vi "Rolling Display.vi"(6 "Input Data":dbl[][](array[numeric]), 9 "Old Data":dbl[][](array[numeric]), 10 "Sample Rate":i32, 11 "Display Size":T3(ring)) -> ()   [LabVIEW 2014]
panel:
  out "Cluster":T1
  in  "Channels in Use":T2
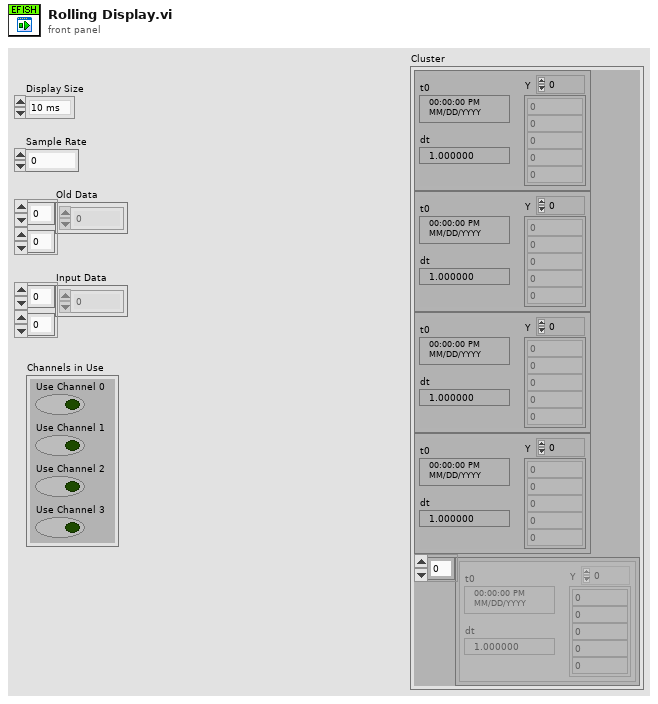
[diagram p1: front panel]
types:
  T1 = cluster{"Waveform":waveform(dbl), "Waveform":waveform(dbl), "Waveform":waveform(dbl), "Waveform":waveform(dbl), waveform(dbl)[]}
  T2 = cluster{"Use Channel 0":bool, "Use Channel 1":bool, "Use Channel 2":bool, "Use Channel 3":bool}
  T3 = enum16{"10 ms", "100 ms", "1 Second", "10 sec", "30 sec"}
  T4 = cluster{waveform(dbl), waveform(dbl), waveform(dbl), waveform(dbl), waveform(dbl)[]}
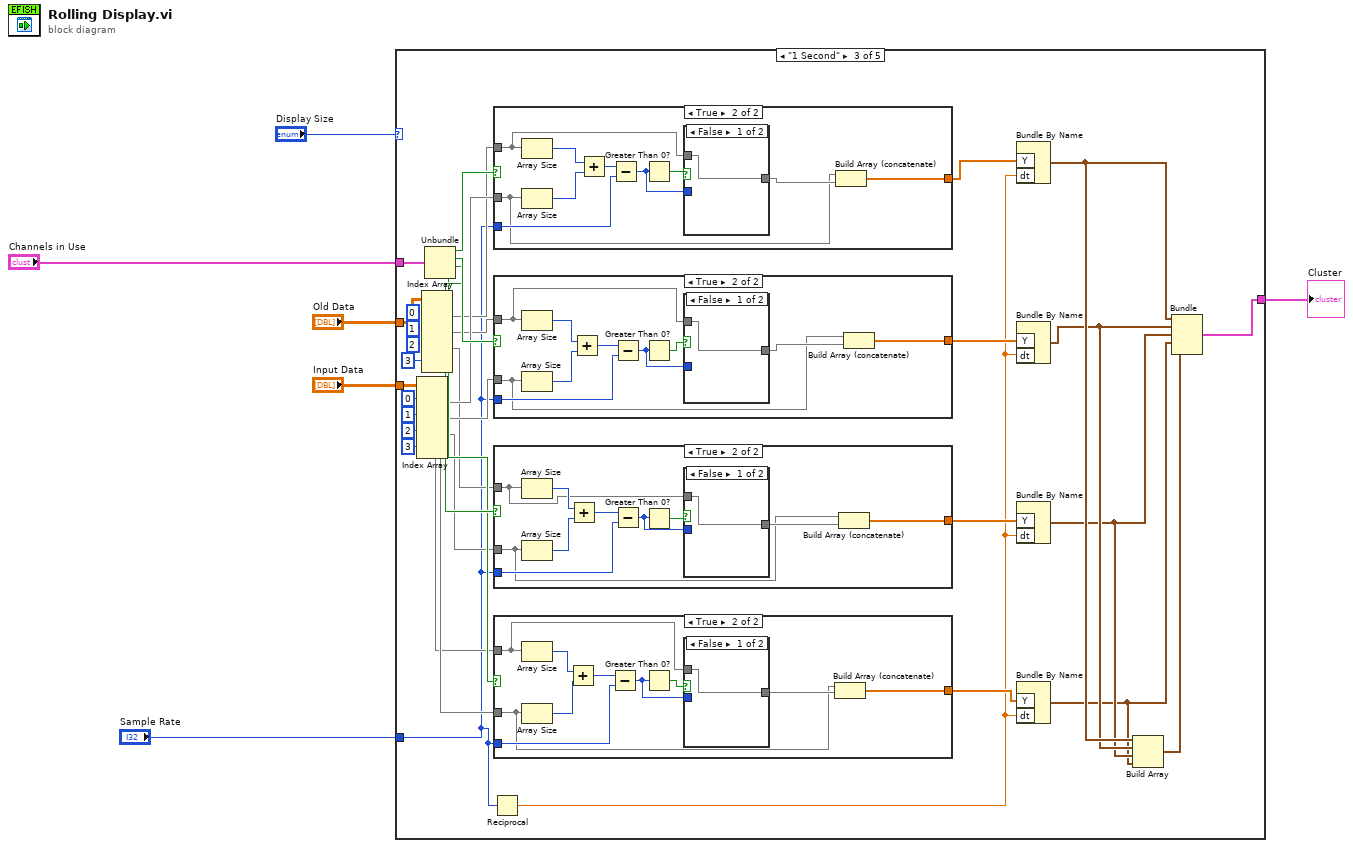
[diagram p0: block diagram]
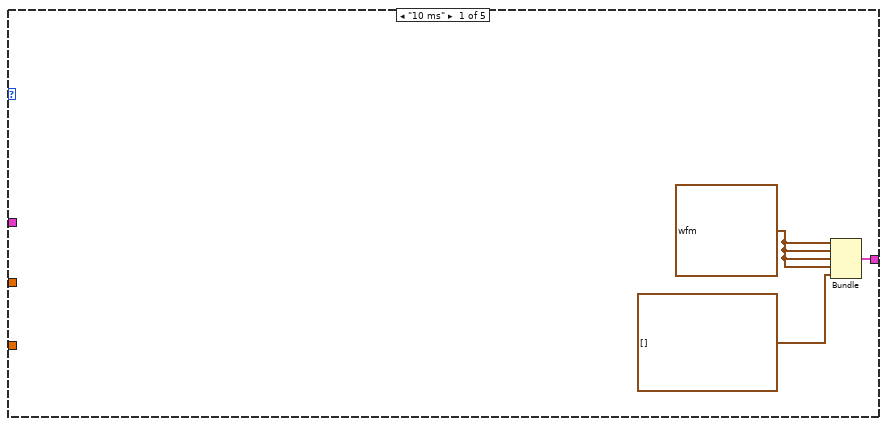
[diagram p2: hidden frame]
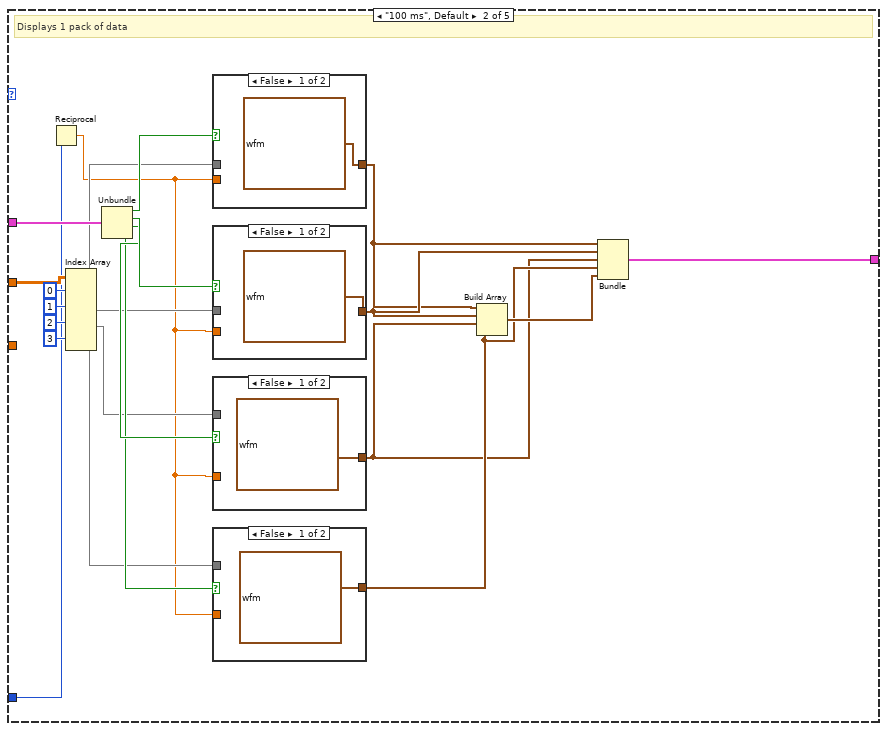
[diagram p3: hidden frame]
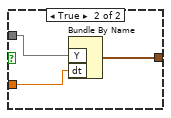
[diagram p4: hidden frame]
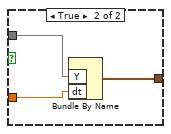
[diagram p5: hidden frame]
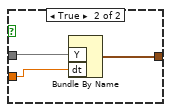
[diagram p6: hidden frame]
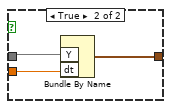
[diagram p7: hidden frame]
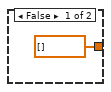
[diagram p8: hidden frame]
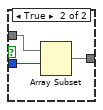
[diagram p9: hidden frame]
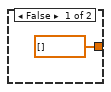
[diagram p10: hidden frame]
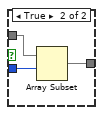
[diagram p11: hidden frame]
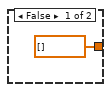
[diagram p12: hidden frame]
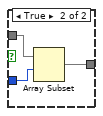
[diagram p13: hidden frame]
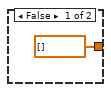
[diagram p14: hidden frame]
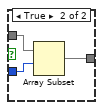
[diagram p15: hidden frame]
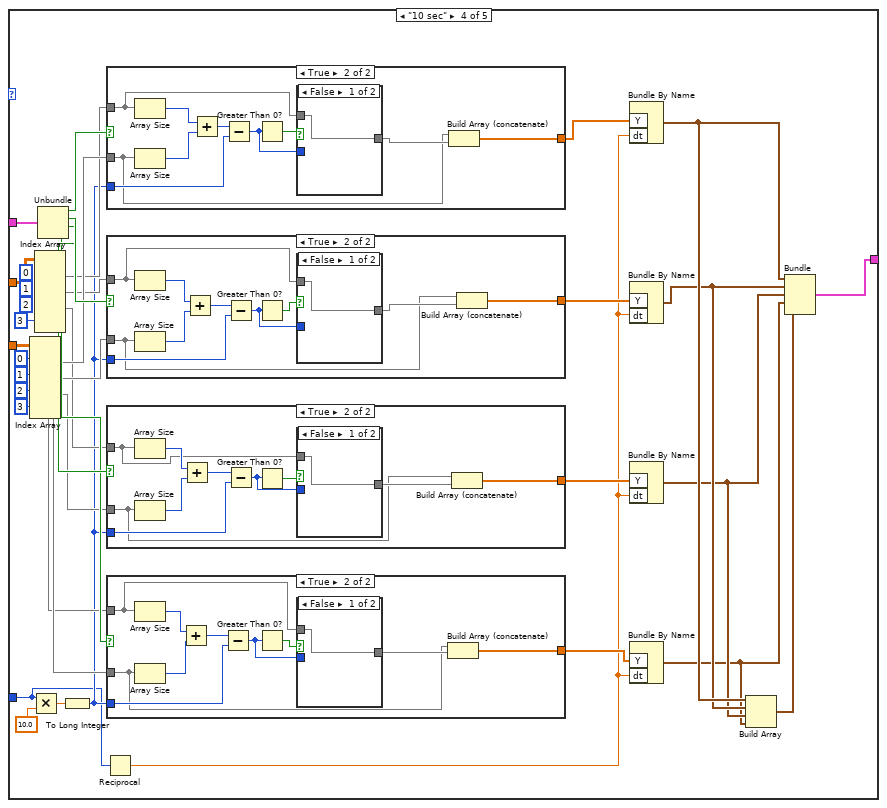
[diagram p16: hidden frame]
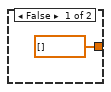
[diagram p17: hidden frame]
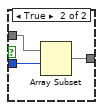
[diagram p18: hidden frame]
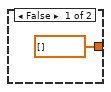
[diagram p19: hidden frame]
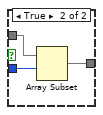
[diagram p20: hidden frame]
diagram:
  n1 = case shown="\"1 Second\"" "Display Size" {
    tunnel: "Sample Rate" -> [_ w17 w48 w147 w242]
    tunnel: "Input Data" -> [_ _ w74 w169 w264]
    tunnel: "Old Data" -> [_ w26 w64 w159 w254]
    tunnel: "Channels in Use" -> [_ w31 w79 w174 w269]
    tunnel: [w9 w10 w49 w140 w235] -> w1
    frame "10 ms" {
      w8 = waveform(dbl) {"t0"=timestamp(0 s since 1904-01-01), "dt"=1.0, "Y"=[]}
      n2 = Bundle(w8, w8, w8, w8, waveform(dbl)[] []) -> (w9:T4)  [unwired: 1 in]
    }
    frame "100 ms", Default {
      # "Displays 1 pack of data"
      n3 = Reciprocal(x=w17) -> (1/x=w16:dbl)
      n4 = Index Array(array=w26, index (row) #1=0 ("index (row)"), index (row) #2=1 ("index (row)"), index (row) #3=2 ("index (row)"), index (row) #4=3 ("index (row)")) -> (element #1=w21:dbl[], element #2=w20:dbl[], element #3=w19:dbl[], element #4=w18:dbl[])  [unwired: 4 in]
      n5 = Unbundle(w31) -> ("Use Channel 0"=w30:bool, "Use Channel 1"=w29:bool, "Use Channel 2"=w28:bool, "Use Channel 3"=w27:bool)
      n6 = case shown="False" w30 {
        tunnel: w21 -> [_ w47]
        tunnel: w16 -> [_ w46]
        tunnel: [waveform(dbl) {"t0"=timestamp(0 s since 1904-01-01), "dt"=1.0, "Y"=[]} w45] -> w11
        frame False {
        }
        frame True {
          n7 = Bundle By Name("Y"=w47, "dt"=w46) -> (w45:waveform(dbl))  [unwired: 1 in]
        }
      }
      n8 = case shown="False" w29 {
        tunnel: w20 -> [_ w43]
        tunnel: w16 -> [_ w42]
        tunnel: [waveform(dbl) {"t0"=timestamp(0 s since 1904-01-01), "dt"=1.0, "Y"=[]} w41] -> w12
        frame False {
        }
        frame True {
          n9 = Bundle By Name("Y"=w43, "dt"=w42) -> (w41:waveform(dbl))  [unwired: 1 in]
        }
      }
      n10 = case shown="False" w28 {
        tunnel: w19 -> [_ w38]
        tunnel: w16 -> [_ w39]
        tunnel: [waveform(dbl) {"t0"=timestamp(0 s since 1904-01-01), "dt"=1.0, "Y"=[]} w37] -> w13
        frame False {
        }
        frame True {
          n11 = Bundle By Name("Y"=w38, "dt"=w39) -> (w37:waveform(dbl))  [unwired: 1 in]
        }
      }
      n12 = case shown="False" w27 {
        tunnel: w18 -> [_ w35]
        tunnel: w16 -> [_ w34]
        tunnel: [waveform(dbl) {"t0"=timestamp(0 s since 1904-01-01), "dt"=1.0, "Y"=[]} w33] -> w14
        frame False {
        }
        frame True {
          n13 = Bundle By Name("Y"=w35, "dt"=w34) -> (w33:waveform(dbl))  [unwired: 1 in]
        }
      }
      n14 = Build Array(w11, w12, w13, w14) -> (w15:waveform(dbl)[])
      n15 = Bundle(w11, w12, w13, w14, w15) -> (w10:T4)  [unwired: 1 in]
    }
    frame "1 Second" {
      (unwired) 2 ("index (row)")
      (unwired) 1 ("index (row)")
      (unwired) 0 ("index (row)")
      n16 = Index Array(array=w74, index (row) #1=0 ("index (row)"), index (row) #2=1 ("index (row)"), index (row) #3=2 ("index (row)"), index (row) #4=3 ("index (row)")) -> (element #1=w69:dbl[], element #2=w68:dbl[], element #3=w67:dbl[], element #4=w66:dbl[])  [unwired: 4 in]
      n17 = Index Array(array=w64, index (row) #4=3 ("index (row)")) -> (element #1=w63:dbl[], element #2=w62:dbl[], element #3=w61:dbl[], element #4=w60:dbl[])  [unwired: 7 in]
      n18 = Unbundle(w79) -> ("Use Channel 0"=w78:bool, "Use Channel 1"=w77:bool, "Use Channel 2"=w76:bool, "Use Channel 3"=w75:bool)
      n19 = Reciprocal(x=w48) -> (1/x=w55:dbl)
      n20 = case shown="True" w78 {
        tunnel: w69 -> [_ w127]
        tunnel: w63 -> [_ w129]
        tunnel: w48 -> [_ w132]
        tunnel: [dbl[] [] w126] -> w59
        frame False {
        }
        frame True {
          n21 = Array Size(array=w129) -> (size(s)=w135:i32)
          n22 = Array Size(array=w127) -> (size(s)=w134:i32)
          n23 = Add(x=w135, y=w134) -> (x+y=w133:i32)
          n24 = Subtract(x=w133, y=w132) -> (x-y=w130:i32)
          n25 = Greater Than 0?(x=w130) -> (x > 0?=w131:bool)
          n26 = case shown="False" w131 {
            tunnel: w130 -> [_ w139]
            tunnel: w129 -> [w136 w138]
            tunnel: [w136 w137] -> w128
            frame False {
            }
            frame True {
              n27 = Array Subset(array=w138, index=w139) -> (w137:dbl[])  [unwired: 1 in]
            }
          }
          n28 = Build Array (concatenate)(w127, w128) -> (w126:dbl[])
        }
      }
      n29 = case shown="True" w77 {
        tunnel: w68 -> [_ w112]
        tunnel: w62 -> [_ w114]
        tunnel: w48 -> [_ w117]
        tunnel: [dbl[] [] w111] -> w58
        frame False {
        }
        frame True {
          n30 = Array Size(array=w114) -> (size(s)=w120:i32)
          n31 = Array Size(array=w112) -> (size(s)=w119:i32)
          n32 = Add(x=w120, y=w119) -> (x+y=w118:i32)
          n33 = Subtract(x=w118, y=w117) -> (x-y=w115:i32)
          n34 = Greater Than 0?(x=w115) -> (x > 0?=w116:bool)
          n35 = case shown="False" w116 {
            tunnel: w115 -> [_ w124]
            tunnel: w114 -> [w121 w123]
            tunnel: [w121 w122] -> w113
            frame False {
            }
            frame True {
              n36 = Array Subset(array=w123, index=w124) -> (w122:dbl[])  [unwired: 1 in]
            }
          }
          n37 = Build Array (concatenate)(w112, w113) -> (w111:dbl[])
        }
      }
      n38 = case shown="True" w76 {
        tunnel: w67 -> [_ w97]
        tunnel: w61 -> [_ w99]
        tunnel: w48 -> [_ w102]
        tunnel: [dbl[] [] w96] -> w57
        frame False {
        }
        frame True {
          n39 = Array Size(array=w99) -> (size(s)=w105:i32)
          n40 = Array Size(array=w97) -> (size(s)=w104:i32)
          n41 = Add(x=w105, y=w104) -> (x+y=w103:i32)
          n42 = Subtract(x=w103, y=w102) -> (x-y=w100:i32)
          n43 = Greater Than 0?(x=w100) -> (x > 0?=w101:bool)
          n44 = case shown="False" w101 {
            tunnel: w100 -> [_ w109]
            tunnel: w99 -> [w106 w108]
            tunnel: [w106 w107] -> w98
            frame False {
            }
            frame True {
              n45 = Array Subset(array=w108, index=w109) -> (w107:dbl[])  [unwired: 1 in]
            }
          }
          n46 = Build Array (concatenate)(w97, w98) -> (w96:dbl[])
        }
      }
      n47 = case shown="True" w75 {
        tunnel: w66 -> [_ w82]
        tunnel: w60 -> [_ w84]
        tunnel: w48 -> [_ w87]
        tunnel: [dbl[] [] w81] -> w56
        frame False {
        }
        frame True {
          n48 = Array Size(array=w84) -> (size(s)=w90:i32)
          n49 = Array Size(array=w82) -> (size(s)=w89:i32)
          n50 = Add(x=w90, y=w89) -> (x+y=w88:i32)
          n51 = Subtract(x=w88, y=w87) -> (x-y=w85:i32)
          n52 = Greater Than 0?(x=w85) -> (x > 0?=w86:bool)
          n53 = case shown="False" w86 {
            tunnel: w85 -> [_ w94]
            tunnel: w84 -> [w91 w93]
            tunnel: [w91 w92] -> w83
            frame False {
            }
            frame True {
              n54 = Array Subset(array=w93, index=w94) -> (w92:dbl[])  [unwired: 1 in]
            }
          }
          n55 = Build Array (concatenate)(w82, w83) -> (w81:dbl[])
        }
      }
      n56 = Bundle By Name("Y"=w59, "dt"=w55) -> (w54:waveform(dbl))  [unwired: 1 in]
      n57 = Bundle By Name("Y"=w58, "dt"=w55) -> (w53:waveform(dbl))  [unwired: 1 in]
      n58 = Bundle By Name("Y"=w57, "dt"=w55) -> (w52:waveform(dbl))  [unwired: 1 in]
      n59 = Bundle By Name("Y"=w56, "dt"=w55) -> (w51:waveform(dbl))  [unwired: 1 in]
      n60 = Build Array(w54, w53, w52, w51) -> (w50:waveform(dbl)[])
      n61 = Bundle(w54, w53, w52, w51, w50) -> (w49:T4)  [unwired: 1 in]
    }
    frame "10 sec" {
      (unwired) 2 ("index (row)")
      (unwired) 1 ("index (row)")
      (unwired) 0 ("index (row)")
      n62 = Index Array(array=w169, index (row) #1=0 ("index (row)"), index (row) #2=1 ("index (row)"), index (row) #3=2 ("index (row)"), index (row) #4=3 ("index (row)")) -> (element #1=w164:dbl[], element #2=w163:dbl[], element #3=w162:dbl[], element #4=w161:dbl[])  [unwired: 4 in]
      n63 = Multiply(x=w147, y=10.0) -> (x*y=w153:dbl)
      n64 = Index Array(array=w159, index (row) #4=3 ("index (row)")) -> (element #1=w158:dbl[], element #2=w157:dbl[], element #3=w156:dbl[], element #4=w155:dbl[])  [unwired: 7 in]
      n65 = Unbundle(w174) -> ("Use Channel 0"=w173:bool, "Use Channel 1"=w172:bool, "Use Channel 2"=w171:bool, "Use Channel 3"=w170:bool)
      n66 = To Long Integer(number=w153) -> (32bit integer=w152:i32)
      n67 = Reciprocal(x=w147) -> (1/x=w146:dbl)
      n68 = case shown="True" w173 {
        tunnel: w164 -> [_ w222]
        tunnel: w158 -> [_ w224]
        tunnel: w152 -> [_ w227]
        tunnel: [dbl[] [] w221] -> w151
        frame False {
        }
        frame True {
          n69 = Array Size(array=w224) -> (size(s)=w230:i32)
          n70 = Array Size(array=w222) -> (size(s)=w229:i32)
          n71 = Add(x=w230, y=w229) -> (x+y=w228:i32)
          n72 = Subtract(x=w228, y=w227) -> (x-y=w225:i32)
          n73 = Greater Than 0?(x=w225) -> (x > 0?=w226:bool)
          n74 = case shown="False" w226 {
            tunnel: w225 -> [_ w234]
            tunnel: w224 -> [w231 w233]
            tunnel: [w231 w232] -> w223
            frame False {
            }
            frame True {
              n75 = Array Subset(array=w233, index=w234) -> (w232:dbl[])  [unwired: 1 in]
            }
          }
          n76 = Build Array (concatenate)(w222, w223) -> (w221:dbl[])
        }
      }
      n77 = case shown="True" w172 {
        tunnel: w163 -> [_ w207]
        tunnel: w157 -> [_ w209]
        tunnel: w152 -> [_ w212]
        tunnel: [dbl[] [] w206] -> w150
        frame False {
        }
        frame True {
          n78 = Array Size(array=w209) -> (size(s)=w215:i32)
          n79 = Array Size(array=w207) -> (size(s)=w214:i32)
          n80 = Add(x=w215, y=w214) -> (x+y=w213:i32)
          n81 = Subtract(x=w213, y=w212) -> (x-y=w210:i32)
          n82 = Greater Than 0?(x=w210) -> (x > 0?=w211:bool)
          n83 = case shown="False" w211 {
            tunnel: w210 -> [_ w219]
            tunnel: w209 -> [w216 w218]
            tunnel: [w216 w217] -> w208
            frame False {
            }
            frame True {
              n84 = Array Subset(array=w218, index=w219) -> (w217:dbl[])  [unwired: 1 in]
            }
          }
          n85 = Build Array (concatenate)(w207, w208) -> (w206:dbl[])
        }
      }
      n86 = case shown="True" w171 {
        tunnel: w162 -> [_ w192]
        tunnel: w156 -> [_ w194]
        tunnel: w152 -> [_ w197]
        tunnel: [dbl[] [] w191] -> w149
        frame False {
        }
        frame True {
          n87 = Array Size(array=w194) -> (size(s)=w200:i32)
          n88 = Array Size(array=w192) -> (size(s)=w199:i32)
          n89 = Add(x=w200, y=w199) -> (x+y=w198:i32)
          n90 = Subtract(x=w198, y=w197) -> (x-y=w195:i32)
          n91 = Greater Than 0?(x=w195) -> (x > 0?=w196:bool)
          n92 = case shown="False" w196 {
            tunnel: w195 -> [_ w204]
            tunnel: w194 -> [w201 w203]
            tunnel: [w201 w202] -> w193
            frame False {
            }
            frame True {
              n93 = Array Subset(array=w203, index=w204) -> (w202:dbl[])  [unwired: 1 in]
            }
          }
          n94 = Build Array (concatenate)(w192, w193) -> (w191:dbl[])
        }
      }
      n95 = case shown="True" w170 {
        tunnel: w161 -> [_ w177]
        tunnel: w155 -> [_ w179]
        tunnel: w152 -> [_ w182]
        tunnel: [dbl[] [] w176] -> w148
        frame False {
        }
        frame True {
          n96 = Array Size(array=w179) -> (size(s)=w185:i32)
          n97 = Array Size(array=w177) -> (size(s)=w184:i32)
          n98 = Add(x=w185, y=w184) -> (x+y=w183:i32)
          n99 = Subtract(x=w183, y=w182) -> (x-y=w180:i32)
          n100 = Greater Than 0?(x=w180) -> (x > 0?=w181:bool)
          n101 = case shown="False" w181 {
            tunnel: w180 -> [_ w189]
            tunnel: w179 -> [w186 w188]
            tunnel: [w186 w187] -> w178
            frame False {
            }
            frame True {
              n102 = Array Subset(array=w188, index=w189) -> (w187:dbl[])  [unwired: 1 in]
            }
          }
          n103 = Build Array (concatenate)(w177, w178) -> (w176:dbl[])
        }
      }
      n104 = Bundle By Name("Y"=w151, "dt"=w146) -> (w145:waveform(dbl))  [unwired: 1 in]
      n105 = Bundle By Name("Y"=w150, "dt"=w146) -> (w144:waveform(dbl))  [unwired: 1 in]
      n106 = Bundle By Name("Y"=w149, "dt"=w146) -> (w143:waveform(dbl))  [unwired: 1 in]
      n107 = Bundle By Name("Y"=w148, "dt"=w146) -> (w142:waveform(dbl))  [unwired: 1 in]
      n108 = Build Array(w145, w144, w143, w142) -> (w141:waveform(dbl)[])
      n109 = Bundle(w145, w144, w143, w142, w141) -> (w140:T4)  [unwired: 1 in]
    }
    frame "30 sec" {
      (unwired) 2 ("index (row)")
      (unwired) 1 ("index (row)")
      (unwired) 0 ("index (row)")
      n110 = Index Array(array=w264, index (row) #1=0 ("index (row)"), index (row) #2=1 ("index (row)"), index (row) #3=2 ("index (row)"), index (row) #4=3 ("index (row)")) -> (element #1=w259:dbl[], element #2=w258:dbl[], element #3=w257:dbl[], element #4=w256:dbl[])  [unwired: 4 in]
      n111 = Multiply(x=w242, y=30.0) -> (x*y=w248:dbl)
      n112 = Index Array(array=w254, index (row) #4=3 ("index (row)")) -> (element #1=w253:dbl[], element #2=w252:dbl[], element #3=w251:dbl[], element #4=w250:dbl[])  [unwired: 7 in]
      n113 = Unbundle(w269) -> ("Use Channel 0"=w268:bool, "Use Channel 1"=w267:bool, "Use Channel 2"=w266:bool, "Use Channel 3"=w265:bool)
      n114 = To Long Integer(number=w248) -> (32bit integer=w247:i32)
      n115 = Reciprocal(x=w242) -> (1/x=w241:dbl)
      n116 = case shown="True" w268 {
        tunnel: w259 -> [_ w317]
        tunnel: w253 -> [_ w319]
        tunnel: w247 -> [_ w322]
        tunnel: [dbl[] [] w316] -> w246
        frame False {
        }
        frame True {
          n117 = Array Size(array=w319) -> (size(s)=w325:i32)
          n118 = Array Size(array=w317) -> (size(s)=w324:i32)
          n119 = Add(x=w325, y=w324) -> (x+y=w323:i32)
          n120 = Subtract(x=w323, y=w322) -> (x-y=w320:i32)
          n121 = Greater Than 0?(x=w320) -> (x > 0?=w321:bool)
          n122 = case shown="False" w321 {
            tunnel: w320 -> [_ w329]
            tunnel: w319 -> [w326 w328]
            tunnel: [w326 w327] -> w318
            frame False {
            }
            frame True {
              n123 = Array Subset(array=w328, index=w329) -> (w327:dbl[])  [unwired: 1 in]
            }
          }
          n124 = Build Array (concatenate)(w317, w318) -> (w316:dbl[])
        }
      }
      n125 = case shown="True" w267 {
        tunnel: w258 -> [_ w302]
        tunnel: w252 -> [_ w304]
        tunnel: w247 -> [_ w307]
        tunnel: [dbl[] [] w301] -> w245
        frame False {
        }
        frame True {
          n126 = Array Size(array=w304) -> (size(s)=w310:i32)
          n127 = Array Size(array=w302) -> (size(s)=w309:i32)
          n128 = Add(x=w310, y=w309) -> (x+y=w308:i32)
          n129 = Subtract(x=w308, y=w307) -> (x-y=w305:i32)
          n130 = Greater Than 0?(x=w305) -> (x > 0?=w306:bool)
          n131 = case shown="False" w306 {
            tunnel: w305 -> [_ w314]
            tunnel: w304 -> [w311 w313]
            tunnel: [w311 w312] -> w303
            frame False {
            }
            frame True {
              n132 = Array Subset(array=w313, index=w314) -> (w312:dbl[])  [unwired: 1 in]
            }
          }
          n133 = Build Array (concatenate)(w302, w303) -> (w301:dbl[])
        }
      }
      n134 = case shown="True" w266 {
        tunnel: w257 -> [_ w287]
        tunnel: w251 -> [_ w289]
        tunnel: w247 -> [_ w292]
        tunnel: [dbl[] [] w286] -> w244
        frame False {
        }
        frame True {
          n135 = Array Size(array=w289) -> (size(s)=w295:i32)
          n136 = Array Size(array=w287) -> (size(s)=w294:i32)
          n137 = Add(x=w295, y=w294) -> (x+y=w293:i32)
          n138 = Subtract(x=w293, y=w292) -> (x-y=w290:i32)
          n139 = Greater Than 0?(x=w290) -> (x > 0?=w291:bool)
          n140 = case shown="False" w291 {
            tunnel: w290 -> [_ w299]
            tunnel: w289 -> [w296 w298]
            tunnel: [w296 w297] -> w288
            frame False {
            }
            frame True {
              n141 = Array Subset(array=w298, index=w299) -> (w297:dbl[])  [unwired: 1 in]
            }
          }
          n142 = Build Array (concatenate)(w287, w288) -> (w286:dbl[])
        }
      }
      n143 = case shown="True" w265 {
        tunnel: w256 -> [_ w272]
        tunnel: w250 -> [_ w274]
        tunnel: w247 -> [_ w277]
        tunnel: [dbl[] [] w271] -> w243
        frame False {
        }
        frame True {
          n144 = Array Size(array=w274) -> (size(s)=w280:i32)
          n145 = Array Size(array=w272) -> (size(s)=w279:i32)
          n146 = Add(x=w280, y=w279) -> (x+y=w278:i32)
          n147 = Subtract(x=w278, y=w277) -> (x-y=w275:i32)
          n148 = Greater Than 0?(x=w275) -> (x > 0?=w276:bool)
          n149 = case shown="False" w276 {
            tunnel: w275 -> [_ w284]
            tunnel: w274 -> [w281 w283]
            tunnel: [w281 w282] -> w273
            frame False {
            }
            frame True {
              n150 = Array Subset(array=w283, index=w284) -> (w282:dbl[])  [unwired: 1 in]
            }
          }
          n151 = Build Array (concatenate)(w272, w273) -> (w271:dbl[])
        }
      }
      n152 = Bundle By Name("Y"=w246, "dt"=w241) -> (w240:waveform(dbl))  [unwired: 1 in]
      n153 = Bundle By Name("Y"=w245, "dt"=w241) -> (w239:waveform(dbl))  [unwired: 1 in]
      n154 = Bundle By Name("Y"=w244, "dt"=w241) -> (w238:waveform(dbl))  [unwired: 1 in]
      n155 = Bundle By Name("Y"=w243, "dt"=w241) -> (w237:waveform(dbl))  [unwired: 1 in]
      n156 = Build Array(w240, w239, w238, w237) -> (w236:waveform(dbl)[])
      n157 = Bundle(w240, w239, w238, w237, w236) -> (w235:T4)  [unwired: 1 in]
    }
  }
  "Cluster" <- w1
